vi "Init Actor Core.vi"(8 "error in (no error)":errorcluster, 11 "Measure Object in":refnum<class "LabActor.lvclass">) -> (0 "error out":errorcluster, 3 "Measure Object out":refnum<class "LabActor.lvclass">)   [LabVIEW 2016, in "LabActor.lvclass"]
uses:
  LabActor.lvclass
  C:/github/LabActor/Template Module/Template Module.lvclass
  <vilib>/Utility/miscctls.llb/LVPositionTypeDef.ctl
  <vilib>/Utility/miscctls.llb/LVRectTypeDef.ctl
  Template Module/Template Module.lvclass/Template Module.ctl
  LabActor.lvclass/LabActor.ctl
  Template Module/Read Front Panel ref.vi
  Controllers/Application Controller/Application Controller.lvclass
panel:
  out "Front Panel Window:Panel Bounds":T1
  out "Origin":T2
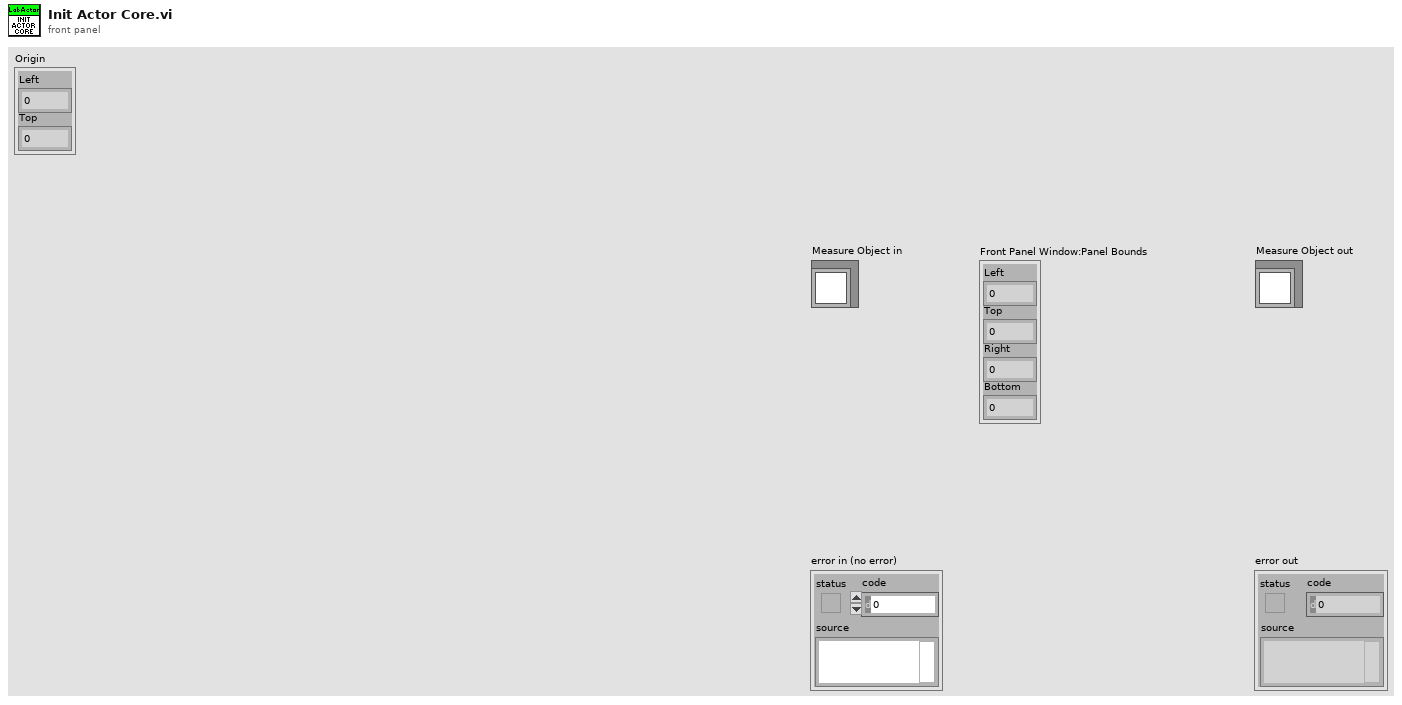
[diagram p1: front panel]
types:
  T1 = typedef "LVRectTypeDef.ctl" = cluster{"Left":i16, "Top":i16, "Right":i16, "Bottom":i16}
  T2 = typedef "LVPositionTypeDef.ctl" = cluster{"Left":i32, "Top":i32}
  T3 = typedef "LVPointTypeDef.ctl" = cluster{"Horizontal":i16, "Vertical":i16}
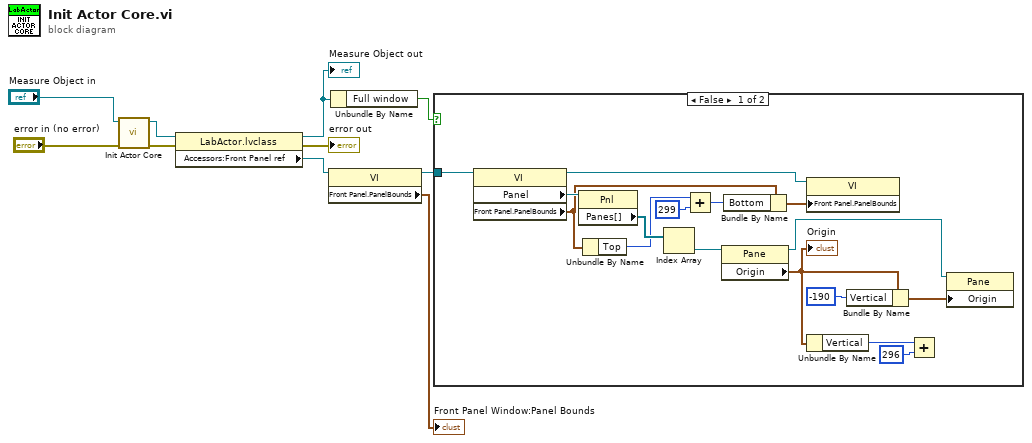
[diagram p0: block diagram]
diagram:
  n1 = call-parent "Init Actor Core.vi"("error in (no error)"="error in (no error)", "Measure Object in"="Measure Object in") -> ("error out"=w10:errorcluster, "Measure Object out"=w5:refnum<class "LabActor.lvclass">)  [unwired: 8 in]
  n2 = property class="LabActor.lvclass"(reference=w5, error in=w10) -> (reference out=w2:refnum<class "LabActor.lvclass">, error out=→"error out":errorcluster, "Accessors:Front Panel ref"=w4:refnum<vi>)
  "Measure Object out" <- w2
  n3 = property class="VI"(reference=w4) -> (reference out=w3:refnum<vi>, "Front Panel.PanelBounds"=→"Front Panel Window:Panel Bounds":T1)  [unwired: 1 in, 1 out]
  n4 = Unbundle By Name(w2) -> ("Full window"=w1:bool)
  n5 = case shown="False" w1 {
    tunnel: w3 -> [w23 _]
    frame False {
      n6 = property class="VI"(reference=w23) -> (reference out=w15:refnum<vi>, "Panel"=w26:refnum<vi>, "Front Panel.PanelBounds"=w18:T1)  [unwired: 1 in, 1 out]
      n7 = property class="Pnl"(reference=w26) -> ("Panes[]"=w25:refnum<vi>[])  [unwired: 1 in, 2 out]
      n8 = Unbundle By Name(w18) -> ("Top"=w13:i16)
      n9 = Index Array(array=w25) -> (element=w24:refnum<vi>)  [unwired: 1 in]
      n10 = Add(x=w13, y=i16 299) -> (x+y=w11:i16)
      n11 = property class="Pane"(reference=w24) -> (reference out=w22:refnum<vi>, "Origin"=w20:T3)  [unwired: 1 in, 1 out]
      "Origin" <- w20
      n12 = Bundle By Name(cluster=w18, "Bottom"=w11) -> (w16:T1)
      n13 = property class="VI"(reference=w15, "Front Panel.PanelBounds"=w16) -> ()  [unwired: 1 in, 2 out]
      n14 = Unbundle By Name(w20) -> ("Vertical"=w21:i16)
      n15 = Bundle By Name(cluster=w20, "Vertical"=i16 -190) -> (w19:T3)
      n16 = Add(x=w21, y=i16 296) -> ()  [unwired: 1 out]
      n17 = property class="Pane"(reference=w22, "Origin"=w19) -> ()  [unwired: 1 in, 2 out]
    }
    frame True {
    }
  }
